vi "Create a New Document.vi"(7 "xwpfDocument Type":refnum<class "xwpfDocument.lvclass">, 8 "error in (no error)":errorcluster, 11 "Document Path":path) -> (0 "error out":errorcluster, 3 "xwpfDocument out":refnum<class "xwpfDocument.lvclass">)   [LabVIEW 2017, in "Word_Specific.lvlib" / "xwpfDocument.lvclass"]
uses:
  xwpfDocument.lvclass
  C:/Users/Neo/Desktop/Dev_Tools_BR/LabVIEW_NPOI/lib/NPOI 2.1.1/NPOI.OOXML.dll
  lib/NPOI 2.1.1/NPOI.OOXML.dll
  xwpfDocument.lvclass/xwpfDocument.ctl
  Support/File Stream/File Stream.lvlib
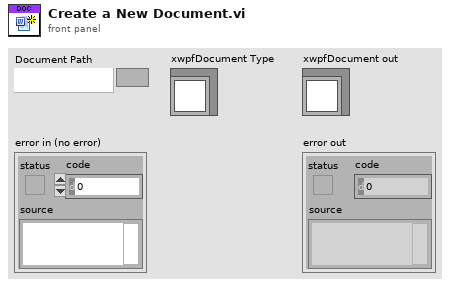
[diagram p1: front panel]
types:
  T1 = enum16{"Title", "Heading 1", "Heading 2", "Heading 3", "Normal", "Figure", "Page Break"}
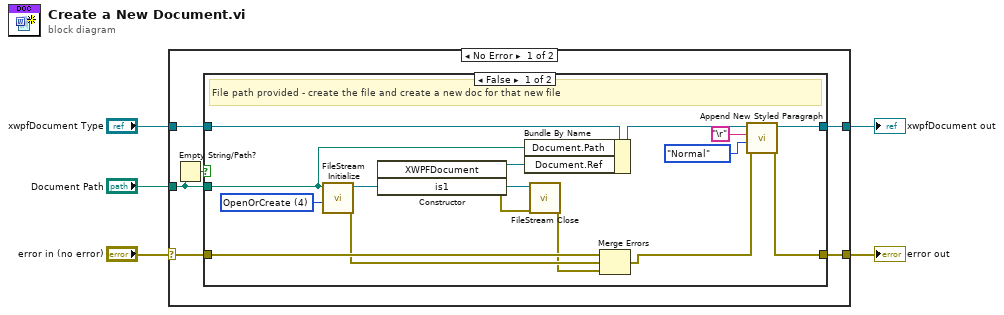
[diagram p0: block diagram]
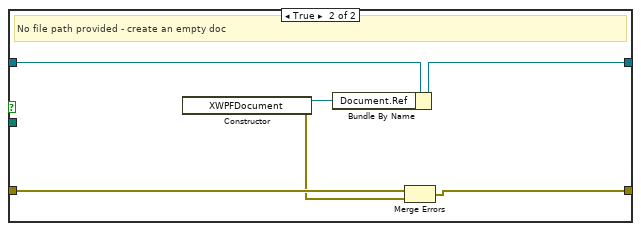
[diagram p2: hidden frame]
diagram:
  n1 = case shown="No Error" "error in (no error)" {
    selector: "error in (no error)" -> [w10 w34]
    tunnel: [w8 w34] -> w2
    tunnel: [w9 w33] -> w4
    tunnel: "xwpfDocument Type" -> [w11 w33]
    tunnel: "Document Path" -> [w7 _]
    frame No Error {
      n2 = Empty String/Path?(string/path=w7) -> (empty?=w6:bool)
      n3 = case shown="False" w6 {
        tunnel: w11 -> [w26 w32]
        tunnel: w10 -> [w25 w31]
        tunnel: [w16 w30] -> w9
        tunnel: [w14 w28] -> w8
        tunnel: w7 -> [w18 _]
        frame False {
          w24 = 4 items=["CreateNew"=1, "Create"=2, "Open"=3, "OpenOrCreate"=4, "Truncate"=5, "Append"=6] ("mode")
          # "File path provided - create the file and create a new doc for that new file"
          n4 = call "FileStream Initialize.vi"("mode"=w24, "path"=w18) -> ("error out"=w20:errorcluster, "new reference"=w22:refnum<k24>)  [unwired: 8 in]
          n5 = constructor class="XWPFDocument"("is1"=w22) -> (reference out=w23:refnum<k24>, error out=w21:errorcluster)  [unwired: 3 in, 2 out]
          n6 = Bundle By Name(cluster=w26, "Document.Path"=w18, "Document.Ref"=w23) -> (w17:refnum<class "xwpfDocument.lvclass">)
          n7 = call "FileStream Close.vi"("error in (no error)"=w21, "reference"=w22) -> ("error out"=w19:errorcluster)  [unwired: 9 in]
          n8 = Merge Errors(w25, w20, w19) -> (w15:errorcluster)
          n9 = call "Append New Styled Paragraph.vi"("error in (no error)"=w15, "Type"=T1."Normal", "Paragraph.Text"="\r", "xwpfDocument in"=w17) -> ("error out"=w14:errorcluster, "xwpfDocument out"=w16:refnum<class "xwpfDocument.lvclass">)  [unwired: 6 in]
        }
        frame True {
          # "No file path provided - create an empty doc"
          n10 = constructor class="XWPFDocument"() -> (reference out=w29:refnum<k24>, error out=w27:errorcluster)  [unwired: 3 in, 1 out]
          n11 = Bundle By Name(cluster=w32, "Document.Ref"=w29) -> (w30:refnum<class "xwpfDocument.lvclass">)
          n12 = Merge Errors(w31, w27) -> (w28:errorcluster)
        }
      }
    }
    frame Error {
    }
  }
  "error out" <- w2
  "xwpfDocument out" <- w4
